vi "Thermistor Read Example.vi"() -> ()   [LabVIEW 2015, in "LabVIEW Interface for Arduino.lvlib"]
doc: "An example that uses an Arduino to read the temperature from a thermistor. The user is able to select the supply voltage, paired resistance, analog input pin and units (C, F, K)."
uses:
  <vilib>/LabVIEW Interface for Arduino/LabVIEW Interface for Arduino.lvlib
panel:
  in  "Paired Resistance (Ohms)":dbl=10000.0
  out "Temperature":dbl(slide) scale=0.0..100.0
  in  "Units":enum16{"Celsius", "Fahrenheit", "Kelvin"}(ring)
  in  "Thermistor AI Pin":u8=1
  in  "Stop":bool
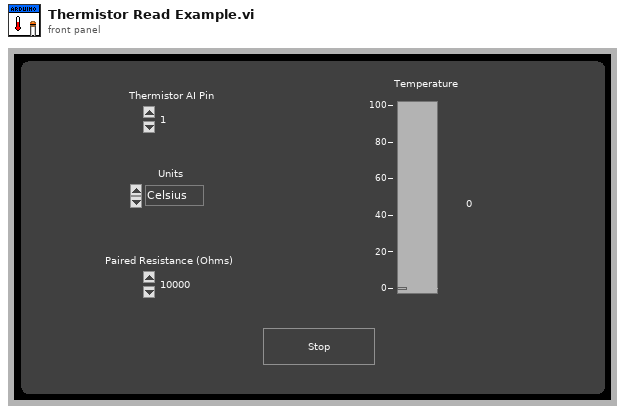
[diagram p1: front panel]
types:
  T1 = typedef "LabVIEW Interface for Arduino.lvlib/Arduino Resource.ctl" = cluster{"VISA resource":refnum<visa-resource-name>, "Board Type":T2, "Connection Type":enum8{"USB / Serial"}, "Bytes Per Packet (15)":u8}
  T2 = typedef "LabVIEW Interface for Arduino.lvlib/Board Type.ctl" = enum16{"Uno", "Dimuelanove w/Atmega 328", "Mega 2560"}
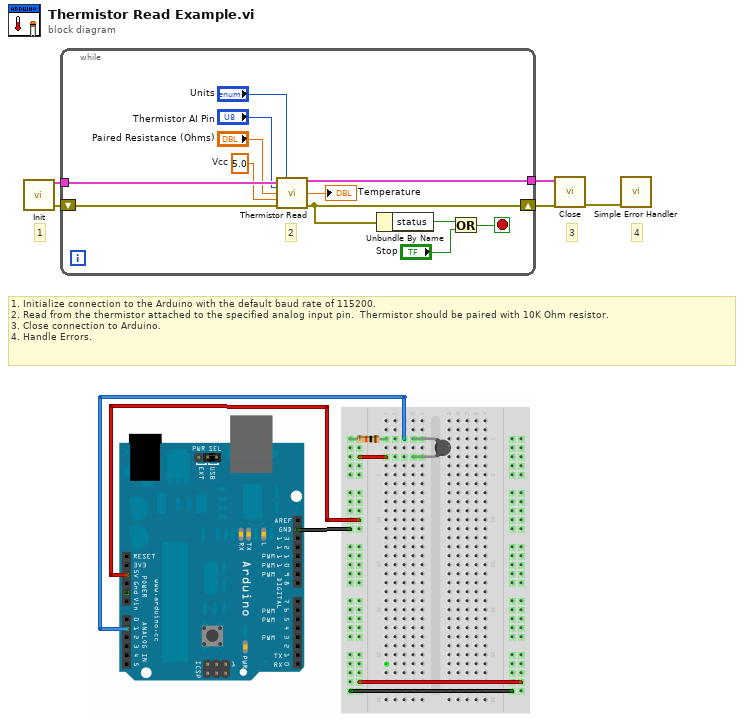
[diagram p0: block diagram]
diagram:
  # "4"
  # "3"
  # "1"
  # "1. Initialize connection to the Arduino with the default baud rate of 115200.\n2. Read from the thermistor attached to the specified analog input pin.  Thermistor should be paired with 10K Ohm resistor.\n3. Close connection to Arduino.\n4. Handle Errors."
  n1 = call <vilib>:"Init.vi"() -> ("Arduino Resource"=w5:T1, "error out"=w4:errorcluster)  [unwired: 18 in]
  n2 = while {
    tunnel: w5 -> [w14]
    shift-right: [w12] -> w2
    shift-left: w4 -> [w13]
    tunnel: [w11] -> w3
    stop <- w15 stop-if-true
    w9 = 5.0  # Vcc
    # "2"
    n3 = call <vilib>:"Thermistor Read.vi"("Arduino Resource"=w14, "Units (C)"="Units", "Thermistor AI Pin (0)"="Thermistor AI Pin", "Paired Resistance (10K Ohms)"="Paired Resistance (Ohms)", "Vcc (5 v)"=w9, "error in"=w13) -> ("Arduino Resource"=w11:T1, "Temperature"=→"Temperature":dbl, "error out"=w12:errorcluster)  [unwired: 7 in]
    n4 = Unbundle By Name(w12) -> ("status"=w17:bool)
    n5 = Or(x=w17, y="Stop") -> (x .or. y?=w15:bool)
  }
  n6 = call <vilib>:"Close.vi"("Arduino Resource"=w3, "error in"=w2) -> ("error out"=w1:errorcluster)  [unwired: 13 in]
  n7 = call <vilib>:"Simple Error Handler.vi"("error in (no error)"=w1) -> ()  [unwired: 4 in, 5 out]
